vi "Get Identifier.vi"(8 "error in":errorcluster, 11 "NI 9862 in":refnum<class "NI 9862.lvclass">) -> (0 "error out":errorcluster, 3 "NI 9862 out":refnum<class "NI 9862.lvclass">)   [LabVIEW 2024, in "NI 9862.lvclass"]
uses:
  NI 9862.lvclass
  NI 9862.lvclass/NI 9862.ctl
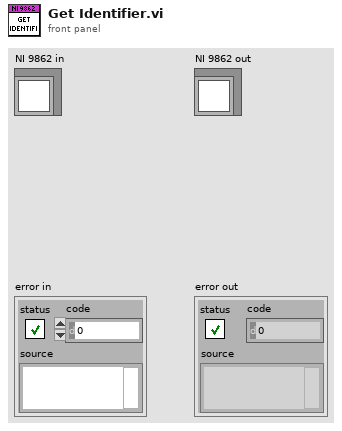
[diagram p1: front panel]
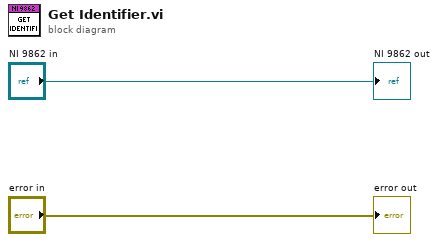
[diagram p0: block diagram]
diagram:
  "error out" <- "error in"
  "NI 9862 out" <- "NI 9862 in"
